vi "UdpServer_KeySim.vi"() -> ()   [LabVIEW 2015]
panel:
  in  "Virtual Key 10":u8(ring)=65
  in  "Virtual Key 9":u8(ring)=65
  out "Up":bool
  out "Down":bool
  in  "Virtual Key 5":u8(ring)=65
  in  "Virtual Key 4":u8(ring)=65
  out "Right":bool
  out "Left":bool
  out "data out":string
  out "port":u16
  out "address":u32
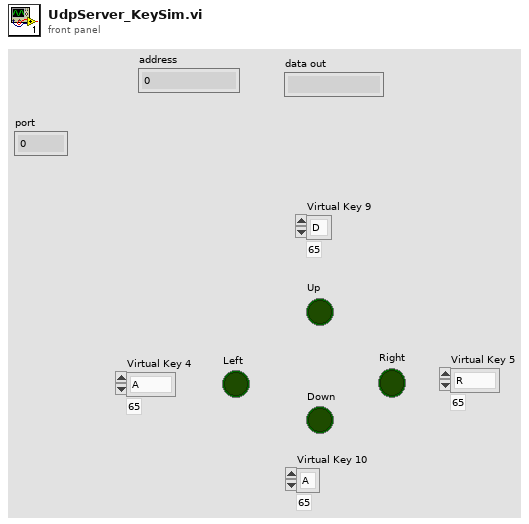
[diagram p1: front panel]
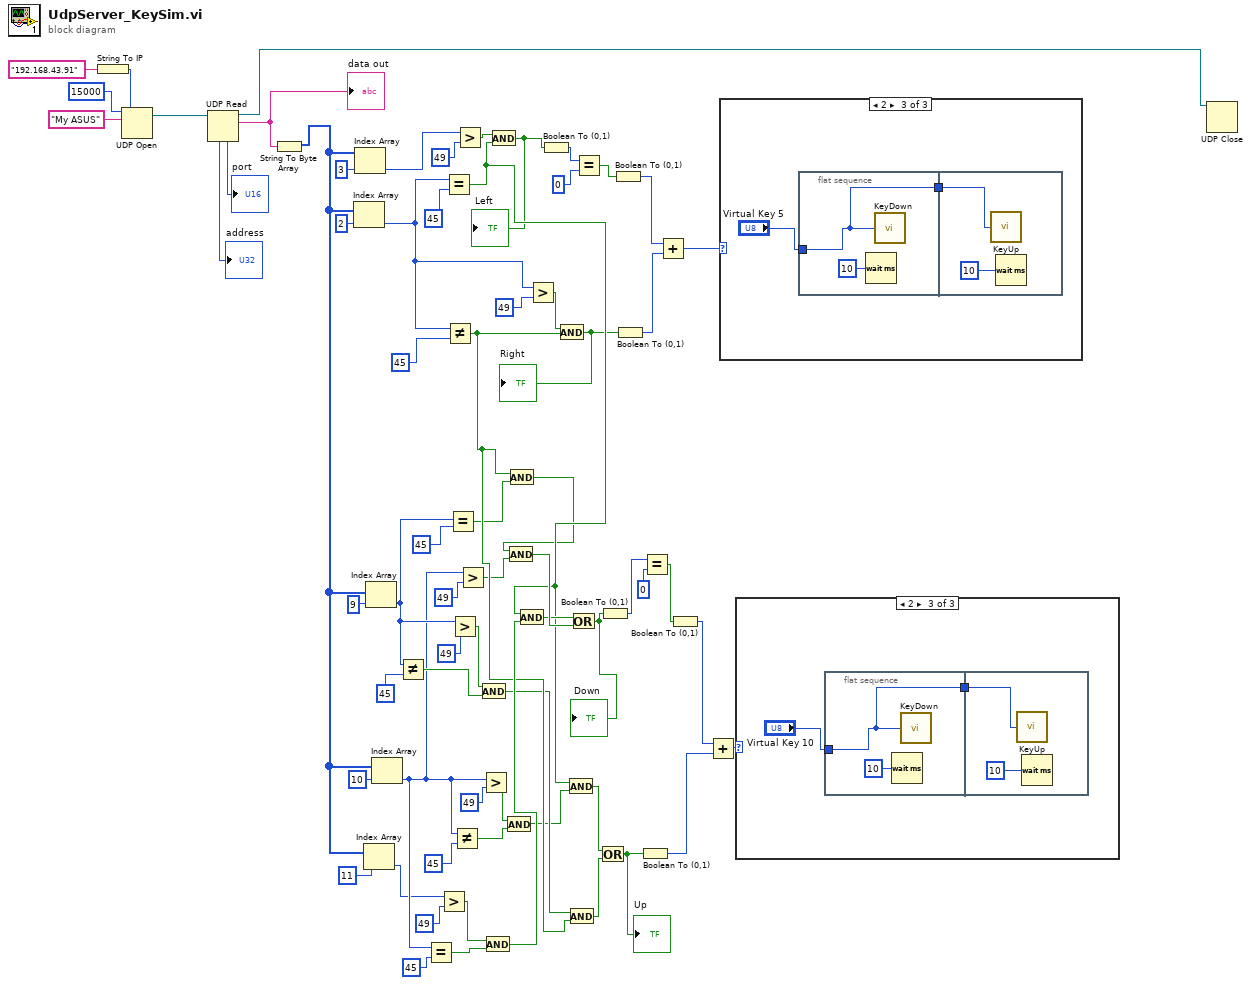
[diagram p0: block diagram]
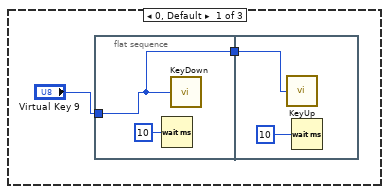
[diagram p2: hidden frame]
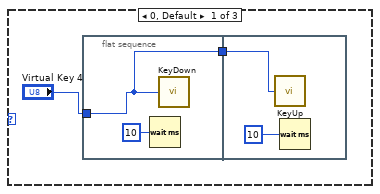
[diagram p4: hidden frame]
diagram:
  n1 = String To IP(1:"192.168.43.91" ("name")) -> (0:w65:u32)
  n2 = UDP Open(7:w65, 10:"My ASUS", 11:u16 15000 ("port")) -> (port=w68:refnum<k16>)  [unwired: 2 in, 2 out]
  n3 = UDP Read(connection ID=w68) -> (data out=w3:string, 3:w63:refnum<k16>, 4:→"port":u16, 6:→"address":u32)  [unwired: 3 in, 1 out]
  "data out" <- w3
  n4 = String To Byte Array(string=w3) -> (unsigned byte array=w37:u8[])
  n5 = Index Array(array=w37, index=2) -> (element=w16:u8)
  n6 = Index Array(array=w37, index=3) -> (element=w10:u8)
  n7 = Index Array(array=w37, index=u8 11 ("y")) -> (element=w40:u8)
  n8 = Index Array(array=w37, index=u8 9 ("y")) -> (element=w51:u8)
  n9 = Index Array(array=w37, index=u8 10 ("y")) -> (element=w43:u8)
  n10 = Not Equal?(x=w51, y=u8 45) -> (x != y?=w53:bool)
  n11 = Equal?(x=w43, y=u8 45) -> (x = y?=w42:bool)
  n12 = Greater?(x=w40, y=49 ("index")) -> (0:w41:bool)
  n13 = Equal?(x=w16, y=u8 45) -> (x = y?=w57:bool)
  n14 = Not Equal?(x=w16, y=u8 45) -> (x != y?=w55:bool)
  n15 = Equal?(x=w51, y=u8 45) -> (x = y?=w33:bool)
  n16 = Greater?(x=w51, y=49 ("index")) -> (0:w52:bool)
  n17 = Not Equal?(x=w43, y=u8 45) -> (x != y?=w35:bool)
  n18 = Greater?(x=w10, y=49 ("index")) -> (0:w9:bool)
  n19 = Greater?(x=w43, y=49 ("index")) -> (0:w26:bool)
  n20 = And(x=w52, y=w53) -> (x .and. y?=w54:bool)
  n21 = Greater?(x=w43, y=49 ("index")) -> (0:w44:bool)
  n22 = And(x=w41, y=w42) -> (x .and. y?=w56:bool)
  n23 = And(x=w9, y=w57) -> (x .and. y?=w22:bool)
  "Left" <- w22
  n24 = And(x=w44, y=w35) -> (x .and. y?=w47:bool)
  n25 = And(x=w55, y=w33) -> (x .and. y?=w34:bool)
  n26 = And(x=w34, y=w26) -> (x .and. y?=w59:bool)
  n27 = And(x=w57, y=w56) -> (x .and. y?=w58:bool)
  n28 = Greater?(x=w16, y=49 ("index")) -> (0:w17:bool)
  n29 = Boolean To (0,1)(Boolean=w22) -> (0, 1=w11:i16)
  n30 = And(x=w17, y=w55) -> (x .and. y?=w23:bool)
  "Right" <- w23
  n31 = And(x=w57, y=w47) -> (x .and. y?=w45:bool)
  n32 = And(x=w54, y=w55) -> (x .and. y?=w46:bool)
  n33 = Or(x=w58, y=w59) -> (x .or. y?=w60:bool)
  "Down" <- w60
  n34 = Equal?(x=w11, y=0 ("index")) -> (x = y?=w13:bool)
  n35 = Or(x=w45, y=w46) -> (x .or. y?=w48:bool)
  "Up" <- w48
  n36 = Boolean To (0,1)(Boolean=w60) -> (0, 1=w27:i16)
  n37 = Boolean To (0,1)(Boolean=w13) -> (0, 1=w14:i16)
  n38 = Boolean To (0,1)(Boolean=w23) -> (0, 1=w18:i16)
  n39 = Boolean To (0,1)(Boolean=w48) -> (0, 1=w32:i16)
  n40 = Equal?(x=w27, y=0 ("index")) -> (x = y?=w61:bool)
  n41 = Add(x=w14, y=w18) -> (x+y=w19:i16)
  n42 = Boolean To (0,1)(Boolean=w61) -> (0, 1=w28:i16)
  n43 = Add(x=w28, y=w32) -> (x+y=w29:i16)
  n44 = case shown="2" w19 {
    frame 0, Default {
      n45 = flat-sequence {
        tunnel: "Virtual Key 4" -> [w71]
        tunnel: [w71] -> w70
        tunnel: w70 -> [w74]
        frame #0 {
          n46 = Wait (ms)(milliseconds to wait=u32 10) -> ()  [unwired: 1 out]
          n47 = call "KeyDown.vi"("Virtual Key"=w71) -> ()  [unwired: 1 in]
        }
        frame #1 {
          n48 = call "KeyUp.vi"("Virtual Key"=w74) -> ()  [unwired: 1 in]
          n49 = Wait (ms)(milliseconds to wait=u32 10) -> ()  [unwired: 1 out]
        }
      }
    }
    frame 1 {
    }
    frame 2 {
      n50 = flat-sequence {
        tunnel: "Virtual Key 5" -> [w77]
        tunnel: [w77] -> w76
        tunnel: w76 -> [w80]
        frame #0 {
          n51 = Wait (ms)(milliseconds to wait=u32 10) -> ()  [unwired: 1 out]
          n52 = call "KeyDown.vi"("Virtual Key"=w77) -> ()  [unwired: 1 in]
        }
        frame #1 {
          n53 = call "KeyUp.vi"("Virtual Key"=w80) -> ()  [unwired: 1 in]
          n54 = Wait (ms)(milliseconds to wait=u32 10) -> ()  [unwired: 1 out]
        }
      }
    }
  }
  n55 = case shown="2" w29 {
    frame 0, Default {
      n56 = flat-sequence {
        tunnel: "Virtual Key 9" -> [w83]
        tunnel: [w83] -> w82
        tunnel: w82 -> [w86]
        frame #0 {
          n57 = Wait (ms)(milliseconds to wait=u32 10) -> ()  [unwired: 1 out]
          n58 = call "KeyDown.vi"("Virtual Key"=w83) -> ()  [unwired: 1 in]
        }
        frame #1 {
          n59 = call "KeyUp.vi"("Virtual Key"=w86) -> ()  [unwired: 1 in]
          n60 = Wait (ms)(milliseconds to wait=u32 10) -> ()  [unwired: 1 out]
        }
      }
    }
    frame 1 {
    }
    frame 2 {
      n61 = flat-sequence {
        tunnel: "Virtual Key 10" -> [w89]
        tunnel: [w89] -> w88
        tunnel: w88 -> [w92]
        frame #0 {
          n62 = Wait (ms)(milliseconds to wait=u32 10) -> ()  [unwired: 1 out]
          n63 = call "KeyDown.vi"("Virtual Key"=w89) -> ()  [unwired: 1 in]
        }
        frame #1 {
          n64 = call "KeyUp.vi"("Virtual Key"=w92) -> ()  [unwired: 1 in]
          n65 = Wait (ms)(milliseconds to wait=u32 10) -> ()  [unwired: 1 out]
        }
      }
    }
  }
  n66 = UDP Close(connection ID=w63) -> ()  [unwired: 1 in, 2 out]
